vi "Handix UI.vi"() -> ()   [LabVIEW 2015]
uses:
  2D Control/2D Buffer Display.xctl
  Instruments/Timothy/FPGA/Rate.ctl
  Instruments/Timothy/CRD/Data/Open Path Data.lvclass
  Instruments/Timothy/CRD/Data/Open Path Data.lvclass/Open Path Data.ctl
  CRDS/Data/Cell/CRDS Cell Data.lvclass/CRDS Cell Data.ctl
  Devices/CR5/Data/CR5 Data.lvclass/CR5 Data.ctl
  Instruments/Timothy/CRD/Data/Read Alicat Data.vi
  Instruments/Timothy/CRD/Data/Accessors/Read CR5.vi
  Instruments/Timothy/CRD/Data/Accessors/Read Heated Line Temp.vi
  Instruments/Timothy/CRD/Data/Accessors/Read Thermistor Data.vi
  Instruments/Timothy/CRD/Data/Accessors/Read u.vi
  Instruments/Timothy/CRD/Data/Accessors/Read VaisalaDuct.vi
  Instruments/Timothy/CRD/Data/Accessors/Read VaisalaOutside.vi
  Instruments/Timothy/CRD/Data/Accessors/Read Pressure.vi
  Devices/CR5/Data/Accessors/Read Balance.vi
  Devices/CR5/Data/Accessors/Read flag.vi
  Devices/CR5/Data/Accessors/Read mirror flag.vi
  Devices/CR5/Data/Accessors/Read PWM.vi
  Devices/CR5/Data/Accessors/Read Tamb.vi
  Devices/CR5/Data/Accessors/Read Tboard.vi
  Devices/CR5/Data/Accessors/Read Tmirror.vi
  CRDS/Data/Cell/Read extParam.vi
  <vilib>/Utility/tcp.llb/UDP Multicast Read-Only Open.vi
  Data/Read measTime.vi
  CRDS/Data/Main/Read CellData.vi
  CRDS/Data/Cell/Read Ringdowns.vi
  CRDS/Data/Cell/CRDS Cell Data.lvclass
  Devices/Alicat/Session Based/Data/Alicat Data.lvclass
  Devices/CR5/Data/CR5 Data.lvclass
panel:
  in  "tabData":enum32{"CRD Output", "IO", "Heater"}(tab)
  out "rdData":i16[][](graph)
  out "derived data":cluster{"data_out":sgl[][], "time":timestamp}(xcontrol)
  in  "connect primary":bool
  out "Pressure":dbl
  in  "Zero State":bool
  in  "Lock":bool=TRUE
  in  "Servo Position (deg)":cluster{u32, u32}(slide)={806, 2337} scale=500.0..2500.0
  in  "Zero (s)":dbl
  in  "Sample (s)":dbl
  in  "cycle?":bool
  in  "Frequency (Hz)":dbl
  in  "Delay (us)":u16=16
  in  "Sample Time (us)":u16=100
  in  "Rate":T1=10 items=["1 MHz"=20, "2 MHz"=10, "2.5 MHz"=8, "5 MHz"=4, "10 MHz"=2, "20MHz"=1]
  in  "# to Coadd":u8=16 min=1 max=50 step=1
  in  "Laser Off (us)":u32=16
  in  "Qpurge (lpm)":cluster{"Sample":sgl, "Zero":sgl} {"Zero" min=0 step=0.01 format="%.2g"; "Sample" min=0 step=0.01 format="%.2g"}
  in  "Invert?":bool
  in  "Bank 1":bool
  in  "Bank 2":bool
  in  "Bank 3":bool
  in  "Primary Volume Fan":dbl(slide) scale=0.0..100.0
  out "Vaisala Duct":cluster{"RH (%)":dbl, "T (degC)":dbl} {"T (degC)" format="%.2f"}
  out "Vaisala Ambient":cluster{"RH (%)":dbl, "T (degC)":dbl} {"T (degC)" format="%.2f"}
  out "Temperature":T2
  out "Duct Velocity":dbl
  out "Alicat Data":T3
  out "CR5 Data":T4
  in  "overrideDeltaT":bool
  in  "delta T":sgl min=0 step=0.01 format="%.2g"
  out "t":T5(graph)
  in  "Tsp":sgl min=0 step=0.01 format="%.2g"
  in  "PID":cluster{"P":sgl, "I":sgl, "D":sgl} {"D" min=0 step=0.01 format="%.2g"; "I" min=0 step=0.01 format="%.2g"; "P" min=0 step=0.01 format="%.2g"}
  in  "heaterPow":bool
  in  "Heater Input":dbl(slide) scale=0.0..100.0
  in  "writeTaus":bool
  out "filtLastSw":timestamp caption="Last Zero" format="%<%H:%M:%S%2u\n%m/%d>T"
  in  "tSwitch":dbl caption="Next Switch (s)"
  in  "newFile":bool
  in  "restart":bool
  in  "SyncTime":bool
  out "Zeroing?":bool
  in  "writeRDs":bool
  out "Version":string
  in  "Save":bool
  out "time":timestamp format="%<%H:%M:%S%2u>T"
  # "CRD Zero"
  # "Open Path CRD Control"
  # "Fan Control"
  # "Laser/Sample Control"
  # "Servo"
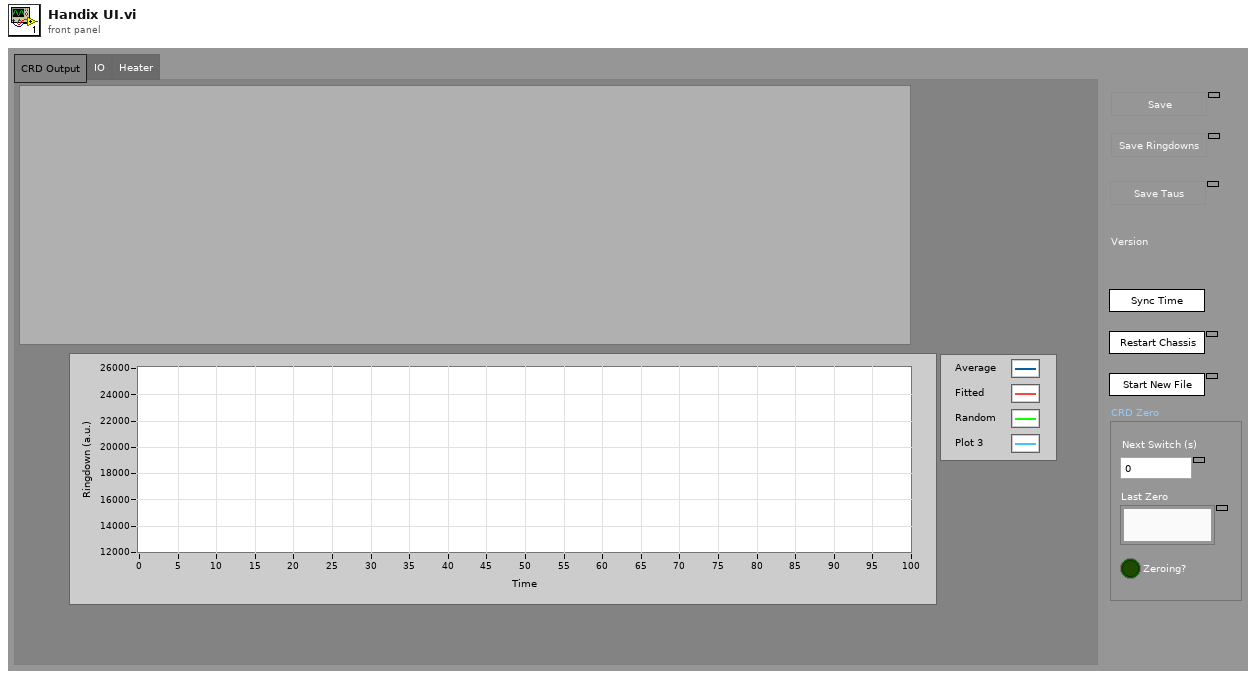
[diagram p1: front panel]
types:
  T1 = typedef "Rate.ctl" = u8
  T2 = cluster{"Thermistor 1":dbl, "Thermistor 2":dbl, "Heated Line":dbl}
  T3 = cluster{"P (mb)":dbl, "T (degC)":dbl, "Q (lpm)":dbl, "Q (slpm)":dbl, "Qsp":dbl}
  T4 = cluster{"Balance":dbl, "Flag":i32, "Mirror Flag":i32, "PWM":dbl, "Tamb (degC)":dbl, "Tboard (degC)":dbl, "Tmirror (degC)":dbl}
  T5 = cluster{"Double":dbl, "Accessors:Heated Line Temp":dbl}
  T6 = cluster{"Read Access":enum8{"Allowed", "Required", "None"}, "Write Access":enum8{"Allowed", "Required", "None"}}
  T7 = cluster{"Name":string, "Line Width":u8, "Line Style":u8, "Color":u32}[]
  T8 = cluster{"Array of Double[0]":dbl, "Array of Double[1]":dbl, "Array of Double[2]":dbl}
  T9 = cluster{"Array of Single[0]":sgl, "Array of Single[1]":sgl}
  T10 = cluster{"Numeric":dbl, "Numeric":dbl, "Accessors:Heated Line Temp":dbl}
  T11 = typedef "extparam.ctl" = cluster{"Tau":sgl, "Tau0cor":sgl, "ext":sgl, "extCorr":sgl, "stdevTau":sgl, "eTau":sgl, "taucorr":sgl, "Tau0":sgl, "max":sgl}
  T12 = cluster{"Accessors:Balance":dbl, "Accessors:flag":i32, "Accessors:mirror flag":i32, "Accessors:PWM":dbl, "Accessors:Tamb":dbl, "Accessors:Tboard":dbl, "Accessors:Tmirror":dbl}
  T13 = cluster{"Accessors:Data[0]":sgl, "Accessors:Data[1]":sgl, "Accessors:Data[2]":sgl, "Accessors:Data[3]":sgl, "Accessors:Data[4]":sgl}
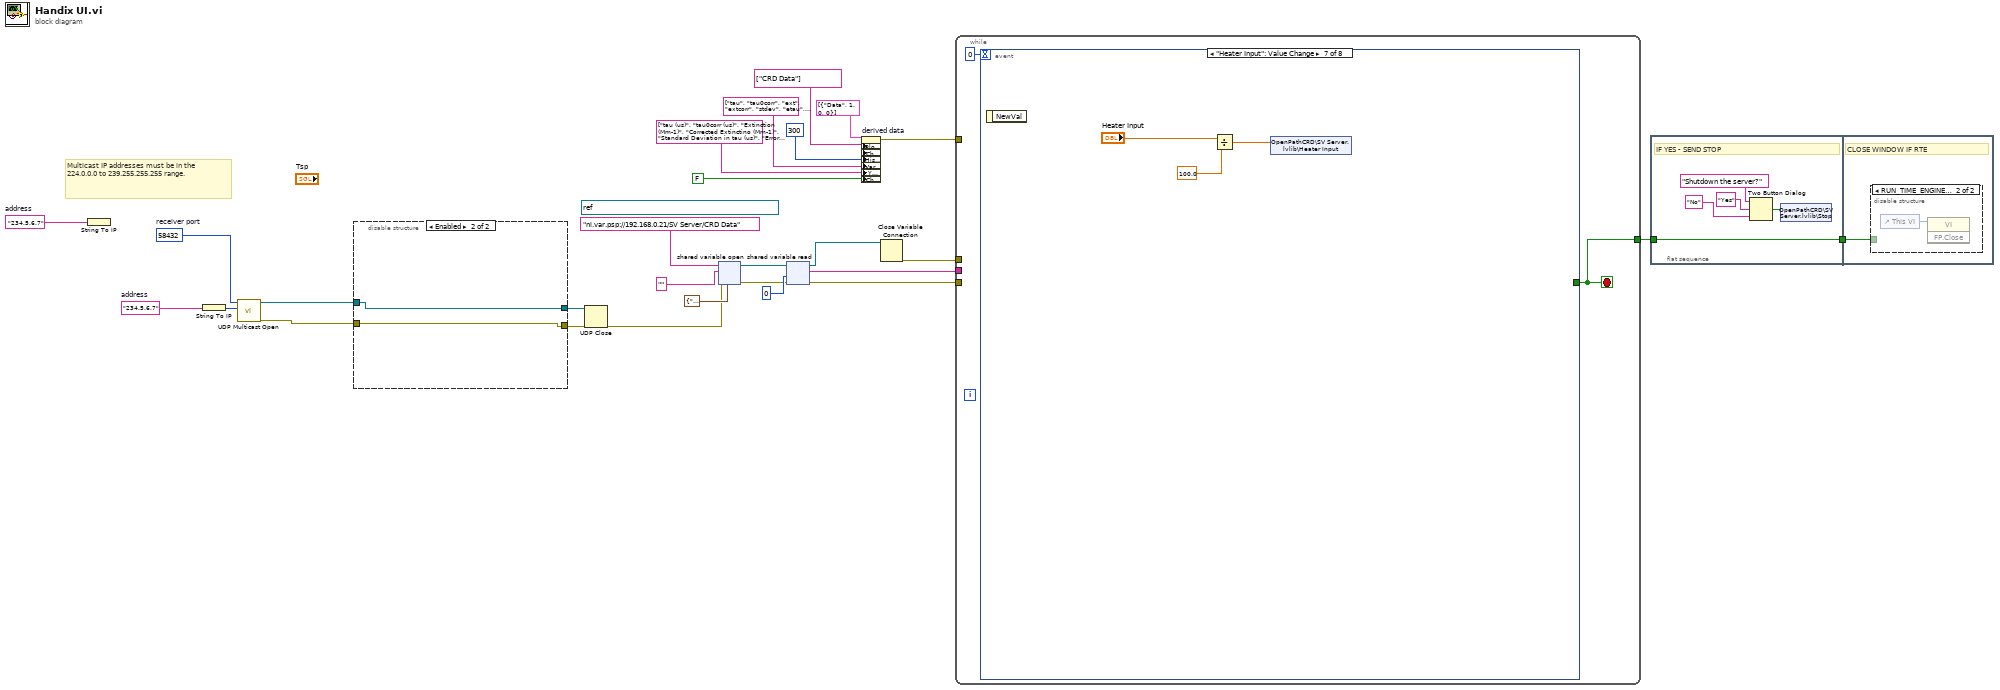
[diagram p0: block diagram]
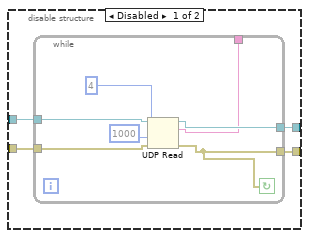
[diagram p2: hidden frame]
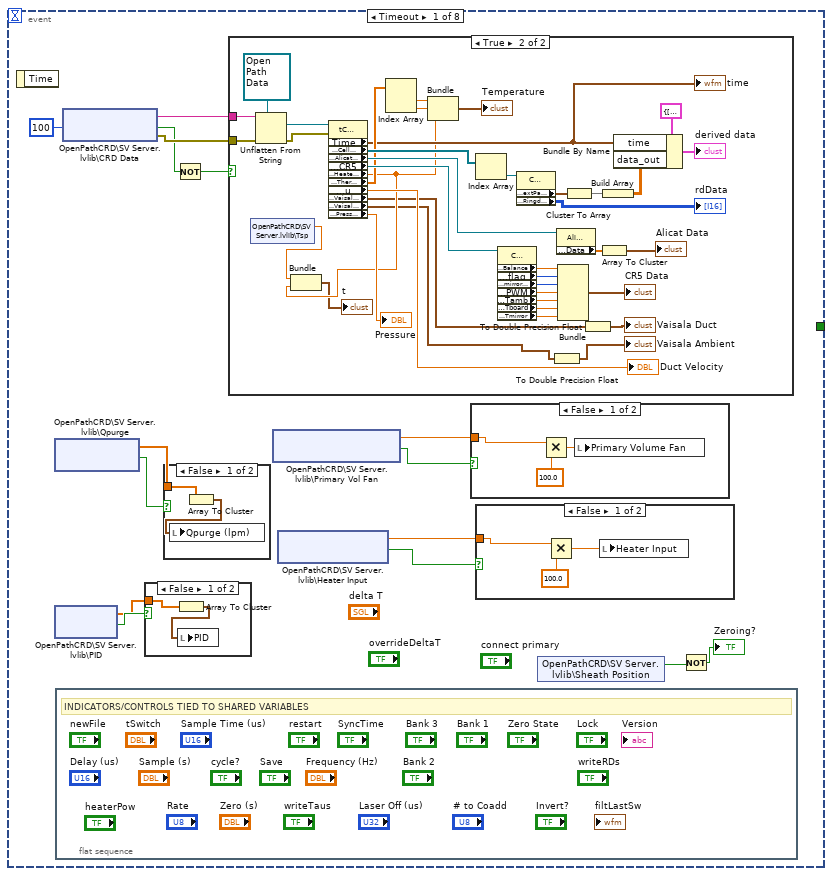
[diagram p4: hidden frame]
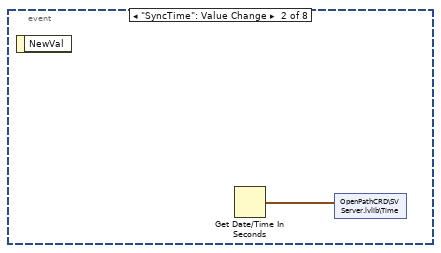
[diagram p10: hidden frame]
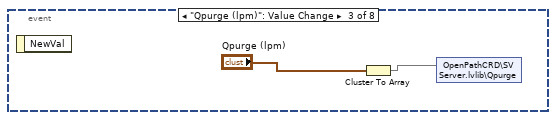
[diagram p11: hidden frame]
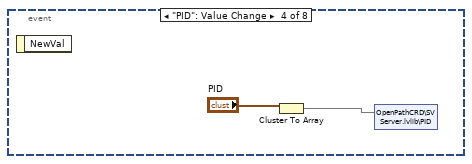
[diagram p12: hidden frame]
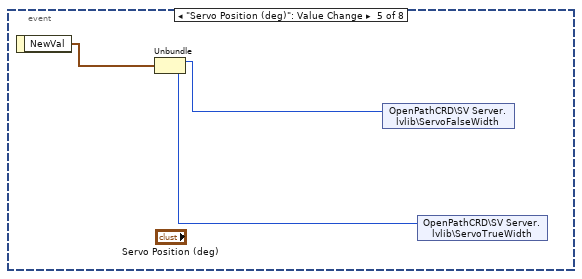
[diagram p13: hidden frame]
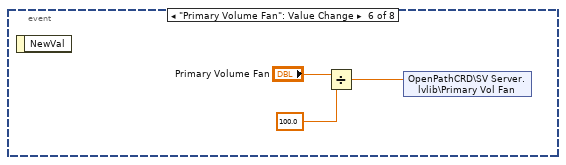
[diagram p14: hidden frame]
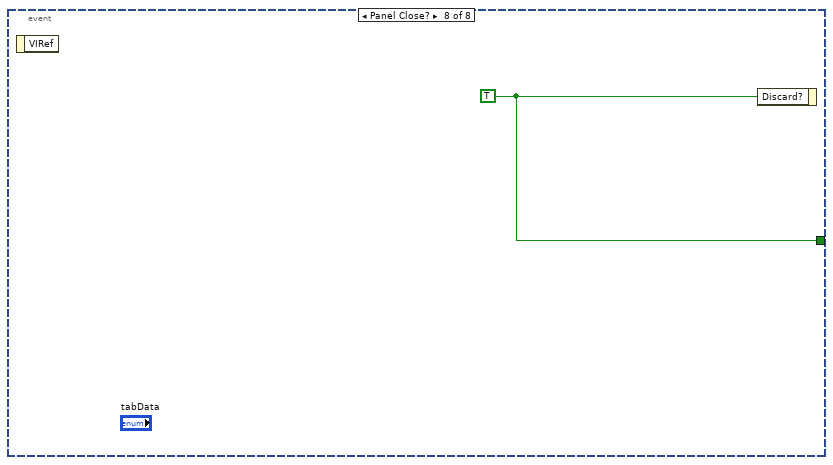
[diagram p15: hidden frame]
diagram:
  w1 = "234.5.6.7"  # address
  w8 = u16 58432  # receiver port
  w9 = "234.5.6.7"  # address
  (unwired) refnum<k21> "ni.var.psp://openpathcrd/SV Server/CRD Data" ("shared variable refnum in")
  # "Multicast IP addresses must be in the 224.0.0.0 to 239.255.255.255 range."
  n1 = String To IP(1:w1) -> ()  [unwired: 1 out]
  n2 = String To IP(1:w9) -> (0:w7:u32)
  n3 = call-poly <vilib>:"UDP Multicast Open.vi"("multicast addr"=w7, "port"=w8) -> ("error out"=w5:errorcluster, "connection ID"=w6:refnum<k16>)  [unwired: 7 in, 1 out]
  n4 = disable-structure shown="Enabled" {
    disable-tunnel: w6 -> [w32 w41]
    disable-tunnel: w5 -> [w31 w40]
    disable-tunnel: [w30 w41] -> w4
    disable-tunnel: [w29 w40] -> w3
    frame Disabled {
      n5 = while {
        tunnel: w32 -> [w38]
        tunnel: w31 -> [w37]
        tunnel: [w36] -> w30
        tunnel: [w35] -> w29
        tunnel: [w34] -> _
        stop <- w35 continue-if-true
        n6 = UDP Read(connection ID=w38, max size (548)=4, timeout ms (25000)=1000, 8:w37) -> (data out=w34:string, error out=w35:errorcluster, 3:w36:refnum<k16>)  [unwired: 2 out]
      }
    }
    frame Enabled {
    }
  }
  n7 = UDP Close(connection ID=w4, 8:w3) -> (error out=w2:errorcluster)  [unwired: 1 out]
  n8 = shared-variable-open("ni.var.psp://192.168.0.21/SV Server/CRD Data", w2, "", T6 {"Read Access"=enum."Allowed", "Write Access"=enum."Allowed"} ("access")) -> (w19:refnum<k21>, w16:errorcluster)
  n9 = shared-variable-read(w19, w16, 0 ("timeout ms")) -> (w12:refnum<k21>, w17:errorcluster, w14:string)  [unwired: 2 out]
  n10 = property on="derived data" class="2D Buffer Display (strict)"("Plot Details"=T7 [{"Name"="Data", "Line Width"=1, "Line Style"=0, "Color"=0}] ("Plot Descr"), "Channels"=string[] ["CRD Data"], "History"=u16 300, "Variables"=string[] ["tau", "tau0corr", "ext", "extcorr", "stdev", "etau", "taucorr", "max"], "Y Axis Labels"=string[] ["tau (us)", "tau0corr (us)", "Extinction (Mm-1)", "Corrected Extinctino (Mm-1)", "Standard Deviation in tau (us)", "Error in Tau", "Corrected tau (us)", "Max Amplitude (a.u.)"] ("Axis Labels"), "Channels Visible?"=FALSE) -> (error out=w23:errorcluster)  [unwired: 2 in, 1 out]
  n11 = Close Variable Connection(11:w12) -> (0:w11:errorcluster)  [unwired: 1 in]
  n12 = while {
    tunnel: w23 -> [_]
    tunnel: [w42] -> w21
    tunnel: w17 -> [_]
    tunnel: w14 -> [_]
    tunnel: w11 -> [_]
    stop <- w42 stop-if-true
    n13 = event shown="[6] \"Heater Input\": Value Change" {
      selector: _ -> [_ _ _ _ _ _ _ _]
      dyn-events: _ -> [_ _ _ _ _ _ _ _]
      timeout: 0 -> [_ _ _ _ _ _ _ _]
      tunnel: [_ _ _ _ _ _ _ w122] -> w42
      event Timeout {
        n14 = event-data() -> ()  [unwired: 1 in, 1 out]
        n15 = shared-variable "OpenPathCRD\\SV Server.lvlib\\Qpurge"() -> (w48:sgl[], w49:bool)  [unwired: 2 in, 1 out]
        n16 = shared-variable "OpenPathCRD\\SV Server.lvlib\\PID"() -> (w46:dbl[], w47:bool)  [unwired: 2 in, 1 out]
        n17 = flat-sequence {
          frame #0 {
            # "INDICATORS/CONTROLS TIED TO SHARED VARIABLES"
          }
        }
        n18 = shared-variable "OpenPathCRD\\SV Server.lvlib\\CRD Data"(100 ("ms timeout (0)")) -> (w58:string, error out=w56:errorcluster, w54:bool)  [unwired: 1 in]
        n19 = case shown="False" w47 {
          tunnel: w46 -> [w60 _]
          frame False {
            n20 = Array To Cluster(array=w60) -> (cluster=w59:T8)
            n21 = local write "PID"(w59) -> ()
          }
          frame True {
          }
        }
        n22 = case shown="False" w49 {
          tunnel: w48 -> [w62 _]
          frame False {
            n23 = Array To Cluster(array=w62) -> (cluster=w61:T9)
            n24 = local write "Qpurge (lpm)"(w61) -> ()
          }
          frame True {
          }
        }
        n25 = Not(x=w54) -> (.not. x?=w55:bool)
        n26 = case shown="True" w55 {
          tunnel: w58 -> [_ w107]
          tunnel: w56 -> [_ w96]
          frame False {
          }
          frame True {
            n27 = shared-variable "OpenPathCRD\\SV Server.lvlib\\Tsp"() -> (w75:dbl)  [unwired: 1 in, 1 out]
            n28 = Unflatten From String(type=refnum<class "Open Path Data.lvclass"> refnum ("tCRD Data"), binary string=w107, error in (no error)=w96) -> (value=w105:refnum<class "Open Path Data.lvclass">, error out=w97:errorcluster)  [unwired: 2 in, 1 out]
            n29 = property class="tCRD Data"(reference=w105, error in=w97) -> ("Time"=w78:timestamp, "Data Access:Cell Data"=w102:refnum<class "CRDS Cell Data.lvclass">[], "Accessors:Alicat Data"=w95:refnum<class "Alicat Data.lvclass">, "Accessors:CR5"=w92:refnum<class "CR5 Data.lvclass">, "Accessors:Heated Line Temp"=w74:dbl, "Accessors:Thermistor Data"=w83:dbl[], "Accessors:u"=→"Duct Velocity":sgl, "Accessors:VaisalaDuct"=w72:cluster{"RH":sgl, "T":sgl}, "Accessors:VaisalaOutside"=w70:cluster{"RH":sgl, "T":sgl}, "Accessors:Pressure"=→"Pressure":dbl)  [unwired: 2 out]
            "time" <- w78
            n30 = Bundle("Double"=w75, "Accessors:Heated Line Temp"=w74) -> (→"t":T5)  [unwired: 1 in]
            n31 = Index Array(array=w83) -> (element #1=w82:dbl, element #2=w81:dbl)  [unwired: 2 in]
            n32 = Bundle("Numeric"=w82, "Numeric"=w81, "Accessors:Heated Line Temp"=w74) -> (→"Temperature":T10)  [unwired: 1 in]
            n33 = Index Array(array=w102) -> (element=w104:refnum<class "CRDS Cell Data.lvclass">)  [unwired: 1 in]
            n34 = property class="CR5 Data"(reference=w92) -> ("Accessors:Balance"=w91:dbl, "Accessors:flag"=w90:i32, "Accessors:mirror flag"=w89:i32, "Accessors:PWM"=w88:dbl, "Accessors:Tamb"=w87:dbl, "Accessors:Tboard"=w86:dbl, "Accessors:Tmirror"=w85:dbl)  [unwired: 1 in, 2 out]
            n35 = property class="CRDS Cell"(reference=w104) -> ("Data Access:extParam"=w103:T11, "Data Access:Ringdowns"=→"rdData":i16[][])  [unwired: 1 in, 2 out]
            n36 = To Double Precision Float(number=w70) -> (double precision float=→"Vaisala Ambient":cluster{"RH":dbl, "T":dbl})
            n37 = property class="Alicat Data"(reference=w95) -> ("Accessors:Data"=w94:sgl[])  [unwired: 1 in, 2 out]
            n38 = Bundle("Accessors:Balance"=w91, "Accessors:flag"=w90, "Accessors:mirror flag"=w89, "Accessors:PWM"=w88, "Accessors:Tamb"=w87, "Accessors:Tboard"=w86, "Accessors:Tmirror"=w85) -> (→"CR5 Data":T12)  [unwired: 1 in]
            n39 = Cluster To Array(cluster=w103) -> (array=w100:sgl[])
            n40 = To Double Precision Float(number=w72) -> (double precision float=→"Vaisala Duct":cluster{"RH":dbl, "T":dbl})
            n41 = Array To Cluster(array=w94) -> (cluster=→"Alicat Data":T13)
            n42 = Build Array(w100) -> (w99:sgl[][])
            n43 = Bundle By Name(cluster=cluster{"data_out":sgl[][], "time":timestamp} {"data_out"=[[0.084651366, 0.25533798, 1.5017034, 2.52959, 3.5592775, 5.9285135, 1.3140382, 3.230594, 3.5457268]], "time"=timestamp(3551230513.8275948 s since 1904-01-01)} ("derived data"), "time"=w78, "data_out"=w99) -> (→"derived data":cluster{"data_out":sgl[][], "time":timestamp})
          }
        }
        n44 = shared-variable "OpenPathCRD\\SV Server.lvlib\\Primary Vol Fan"() -> (w52:dbl, w53:bool)  [unwired: 2 in, 1 out]
        n45 = shared-variable "OpenPathCRD\\SV Server.lvlib\\Heater Input"() -> (w51:dbl, w50:bool)  [unwired: 2 in, 1 out]
        n46 = case shown="False" w53 {
          tunnel: w52 -> [w68 _]
          frame False {
            n47 = Multiply(x=w68, y=100.0) -> (x*y=w66:dbl)
            n48 = local write "Primary Volume Fan"(w66) -> ()
          }
          frame True {
          }
        }
        n49 = case shown="False" w50 {
          tunnel: w51 -> [w65 _]
          frame False {
            n50 = Multiply(x=w65, y=100.0) -> (x*y=w63:dbl)
            n51 = local write "Heater Input"(w63) -> ()
          }
          frame True {
          }
        }
        n52 = shared-variable "OpenPathCRD\\SV Server.lvlib\\Sheath Position"() -> (w45:bool)  [unwired: 1 in, 1 out]
        n53 = Not(x=w45) -> (.not. x?=→"Zeroing?":bool)
      }
      event "SyncTime": Value Change {
        n54 = event-data() -> ()  [unwired: 1 in, 1 out]
        n55 = Get Date/Time In Seconds() -> (seconds since 1Jan1904=w108:timestamp)
        n56 = shared-variable "OpenPathCRD\\SV Server.lvlib\\Time"(w108) -> ()  [unwired: 1 in, 1 out]
      }
      event "Qpurge (lpm)": Value Change {
        n57 = event-data() -> ()  [unwired: 1 in, 1 out]
        n58 = Cluster To Array(cluster="Qpurge (lpm)") -> (array=w109:sgl[])
        n59 = shared-variable "OpenPathCRD\\SV Server.lvlib\\Qpurge"(w109) -> ()  [unwired: 1 in, 1 out]
      }
      event "PID": Value Change {
        n60 = event-data() -> ()  [unwired: 1 in, 1 out]
        n61 = Cluster To Array(cluster="PID") -> (array=w111:sgl[])
        n62 = shared-variable "OpenPathCRD\\SV Server.lvlib\\PID"(w111) -> ()  [unwired: 1 in, 1 out]
      }
      event "Servo Position (deg)": Value Change {
        n63 = event-data() -> ("NewVal"=w115:cluster{u32, u32})  [unwired: 1 in]
        n64 = Unbundle(w115) -> (w114:u32, w113:u32)
        n65 = shared-variable "OpenPathCRD\\SV Server.lvlib\\ServoFalseWidth"(w114) -> ()  [unwired: 1 in, 1 out]
        n66 = shared-variable "OpenPathCRD\\SV Server.lvlib\\ServoTrueWidth"(w113) -> ()  [unwired: 1 in, 1 out]
      }
      event "Primary Volume Fan": Value Change {
        n67 = event-data() -> ()  [unwired: 1 in, 1 out]
        n68 = Divide(x="Primary Volume Fan", y=100.0) -> (x/y=w116:dbl)
        n69 = shared-variable "OpenPathCRD\\SV Server.lvlib\\Primary Vol Fan"(w116) -> ()  [unwired: 1 in, 1 out]
      }
      event "Heater Input": Value Change {
        n70 = event-data() -> ()  [unwired: 1 in, 1 out]
        n71 = Divide(x="Heater Input", y=100.0) -> (x/y=w120:dbl)
        n72 = shared-variable "OpenPathCRD\\SV Server.lvlib\\Heater Input"(w120) -> ()  [unwired: 1 in, 1 out]
      }
      event Panel Close? {
        w122 = TRUE ("Discard?")
        n73 = event-data() -> ()  [unwired: 1 in, 1 out]
        n74 = event-data("Discard?"=w122) -> ()  [unwired: 1 in, 1 out]
      }
    }
  }
  n75 = flat-sequence {
    tunnel: w21 -> [w127]
    tunnel: [w127] -> w20
    tunnel: w20 -> [w128]
    frame #0 {
      # "IF YES - SEND STOP"
      n76 = Two Button Dialog(message="Shutdown the server?", 1:"No" ("F button name (\"Cancel\")"), 2:"Yes" ("T button name (\"OK\")")) -> (T button?=w125:bool)
      n77 = shared-variable "OpenPathCRD\\SV Server.lvlib\\Stop"(w125) -> ()  [unwired: 1 in, 1 out]
    }
    frame #1 {
      # "CLOSE WINDOW IF RTE"
      n78 = disable-structure shown="RUN_TIME_ENGINE==True" {
        disable-tunnel: w128 -> [_ _]
        frame condition #0 (active) {
        }
        frame condition #1 {
          n79 = control-ref of="This VI"() -> (w129:refnum<vi>)
          n80 = invoke class="VI" method="FP.Close"(reference=w129) -> ()  [unwired: 2 in, 3 out]
        }
      }
    }
  }
